vi "CameraSetTrigger.vi"(8 "error in (no error)":errorcluster, 10 "external?":bool=TRUE, 11 "Photonfocus in":refnum<class "Photonfocus.lvclass">) -> (0 "error out":errorcluster, 2 "attribs":variant[](array[variant]), 3 "Photonfocus out":refnum<class "Photonfocus.lvclass">)   [LabVIEW 2010, in "Photonfocus.lvclass"]
uses:
  <userlib>/bias/classes/Photonfocus/Photonfocus.lvclass
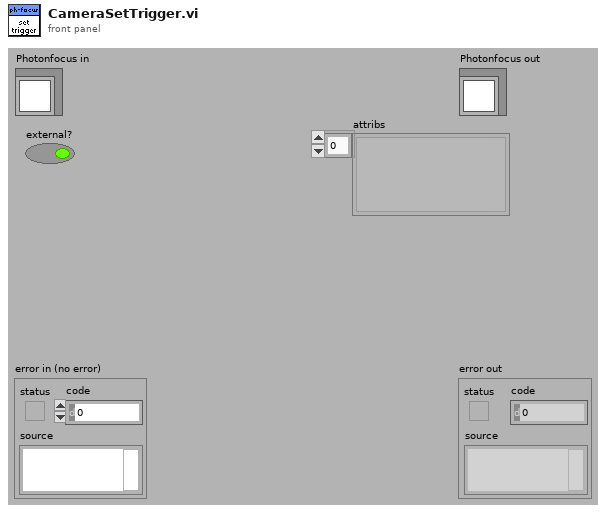
[diagram p1: front panel]
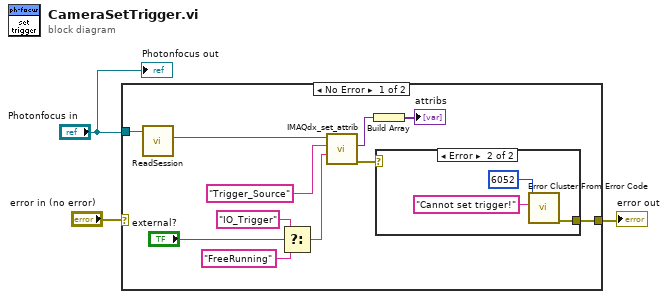
[diagram p0: block diagram]
diagram:
  n1 = case shown="No Error" "error in (no error)" {
    selector: "error in (no error)" -> [_ w18]
    tunnel: [w8 w18] -> w3
    tunnel: "Photonfocus in" -> [w5 _]
    frame No Error {
      n2 = call-dynamic "ReadSession.vi"("IMAQdx in"=w5) -> ("session"=w4:refnum<k21>)  [unwired: 9 in, 1 out]
      n3 = Select(t="IO_Trigger" ("f"), s="external?", f="FreeRunning" ("attribute")) -> (s? t:f=w10:string)
      n4 = call <userlib>:"IMAQdx_set_attrib.vi"("value"=w10, "attribute"="Trigger_Source", "IMAQdx in"=w4) -> ("error out"=w9:errorcluster, "attrib out"=w6:variant)  [unwired: 2 in, 1 out]
      n5 = Build Array(w6) -> (→"attribs":variant[])
      n6 = case shown="Error" w9 {
        tunnel: [_ w17] -> w8
        frame No Error {
        }
        frame Error {
          n7 = call <vilib>:"Error Cluster From Error Code.vi"("error message (\"\")"="Cannot set trigger!" ("error message (\"\")"), "error code (0)"=6052) -> ("error out"=w17:errorcluster)  [unwired: 7 in]
        }
      }
    }
    frame Error {
    }
  }
  "error out" <- w3
  "Photonfocus out" <- "Photonfocus in"
